vi "slowdown function.vi"(4 "max speed":dbl=20000.0, 6 "min speed":dbl=500.0, 8 "update rate":i32=250, 9 "width":dbl=0.1, 10 "threshold":dbl=1.0, 11 "lambda":dbl) -> (3 "freq step":dbl)   [LabVIEW 2010]
panel:
  out "Plot:response":cluster{dbl[], dbl[]}[](graph)
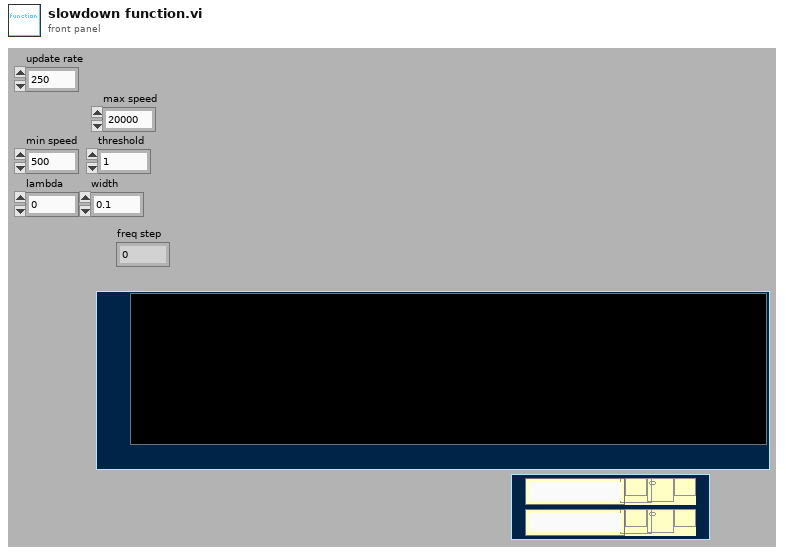
[diagram p1: front panel]
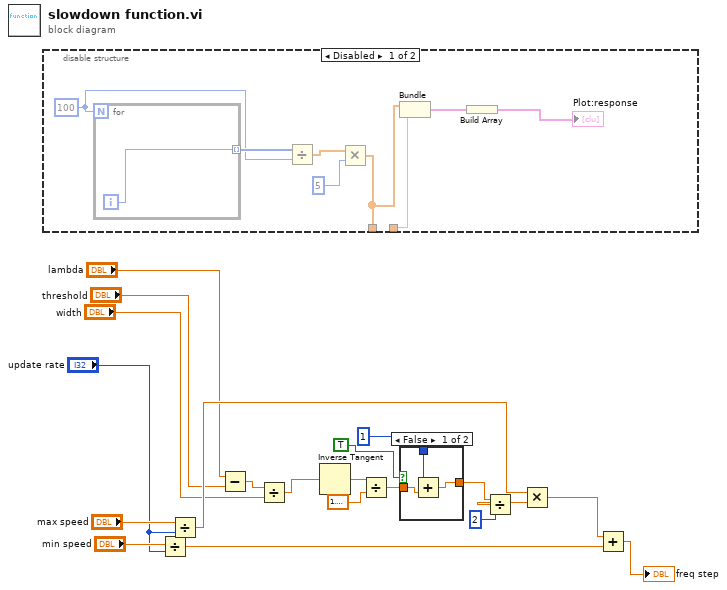
[diagram p0: block diagram]
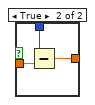
[diagram p2: hidden frame]
diagram:
  n1 = disable-structure shown="Disabled" {
    disable-tunnel: [w22 _] -> _
    disable-tunnel: _ -> [w21 _]
    frame Disabled {
      w27 = 100
      n2 = for {
        N: w27 -> [_]
        tunnel: [w29] -> w28 mode=indexing
        i -> [w29]
      }
      n3 = Divide(x=w28, y=w27) -> (x/y=w26:dbl[])
      n4 = Multiply(x=w26, y=5) -> (x*y=w22:dbl[])
      n5 = Bundle(w22, w21) -> (w24:cluster{dbl[], void})  [unwired: 1 out]
      n6 = Build Array(w24) -> (→"Plot:response":cluster{dbl[], void}[])
    }
    frame Enabled {
    }
  }
  n7 = Divide(x="min speed", y="update rate") -> (x/y=w17:dbl)
  n8 = Divide(x="max speed", y="update rate") -> (x/y=w13:dbl)
  n9 = Subtract(x="lambda", y="threshold") -> (x-y=w9:dbl)
  n10 = Divide(x=w9, y="width") -> (x/y=w7:dbl)
  n11 = Inverse Tangent(1:w7) -> (0:w16:dbl)
  n12 = Divide(x=w16, y=1.5707963267948966) -> (x/y=w4:dbl)
  n13 = case shown="False" TRUE {
    tunnel: [w31 w35] -> w6
    tunnel: 1 -> [w30 w34]
    tunnel: w4 -> [w32 w33]
    frame False {
      n14 = Add(x=w30, y=w32) -> (x+y=w31:dbl)
    }
    frame True {
      n15 = Subtract(x=w34, y=w33) -> (x-y=w35:dbl)
    }
  }
  n16 = Divide(x=w6, y=2) -> (x/y=w12:dbl)
  n17 = Multiply(x=w13, y=w12) -> (x*y=w11:dbl)
  n18 = Add(x=w11, y=w17) -> (x+y=→"freq step":dbl)
